vi "Parse Attribute.vi"(4 "Header Values":string[](array[string]), 6 "Header Names":string[](array[string]), 8 "error in (no error)":errorcluster, 9 "Tag Name":string, 10 "Flattened Linked List":string, 11 "IPersist in":refnum<class "IPersist.lvclass">) -> (0 "error out":errorcluster, 2 "Flattened Linked List out":string, 3 "IPersist out":refnum<class "IPersist.lvclass">, 5 "Attribute Value":variant, 7 "Attribute Name":string)   [LabVIEW 2019, in "IPersist.lvlib" / "IPersist.lvclass"]
uses:
  <vilib>/gpm_packages/@cs/persistence/source/IPersist/IPersist.lvclass
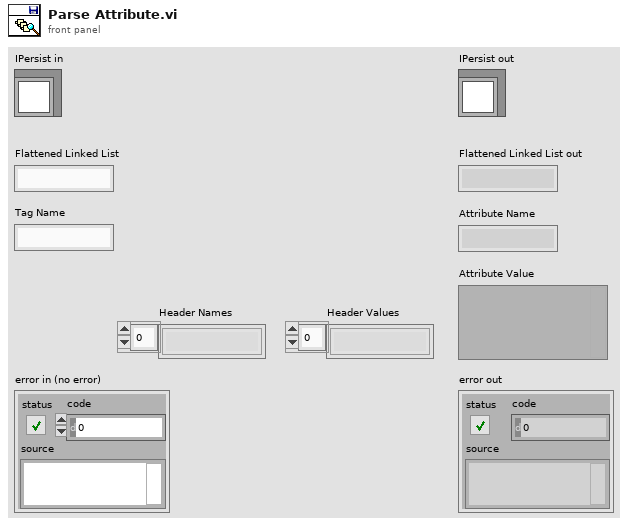
[diagram p1: front panel]
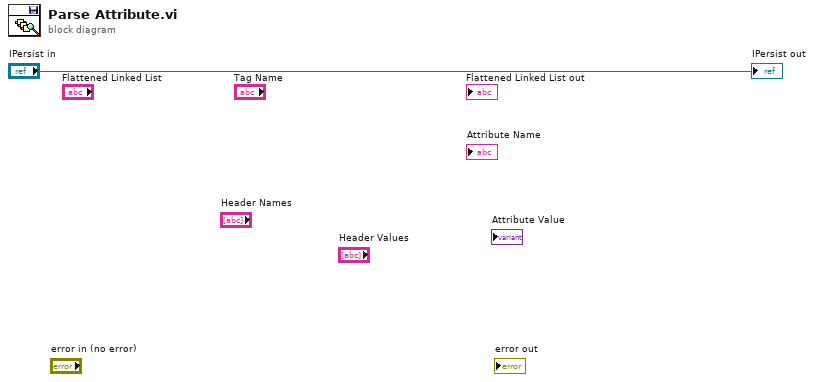
[diagram p0: block diagram]
diagram:
  "IPersist out" <- "IPersist in"
